vi "pmu_Simulate PMU signal.vi"(0 "physical channels":T1[](array[typedef]), 5 "elements to read":u32=250, 7 "frequency (Hz)":dbl(knob)=60.0 scale=45.0..65.0 scale format="%#.9g", 11 "error in (no error)":errorcluster) -> (4 "FIFO data":u32[](array[numeric]), 15 "error out":errorcluster)   [LabVIEW 2014]
doc: "This VI simulates pure sinewave test signal to validate the RT part of the PMU algorithm. You can set frequency, amplitude and digital signal states with this VI. This VI is intended to be used in debugging mode with its front panel open so that the user can control front panel objects."
uses:
  <vilib>/addons/Electrical Power/PMU/Common/Controls/pmu_Physical Channel.ctl
  <vilib>/addons/Electrical Power/PMU/Common/Controls/pmu_Channel Phase.ctl
  <vilib>/addons/Electrical Power/PMU/NI_EP_PMU.lvlib
panel:
  in  "Random DI":bool
  in  "DI":bool[](array[boolean])=[FALSE, FALSE, FALSE, FALSE, FALSE, FALSE, FALSE, FALSE, FALSE, FALSE, FALSE, FALSE, FALSE, FALSE, FALSE, FALSE, FALSE, FALSE, FALSE, FALSE, FALSE, FALSE, FALSE, FALSE, FALSE, FALSE, FALSE, FALSE, FALSE, FALSE, FALSE, FALSE]
  in  "current (A)":dbl(knob)=2.5 scale=0.0..5.0
  in  "voltage (V)":dbl(knob)=110.0 scale=0.0..300.0
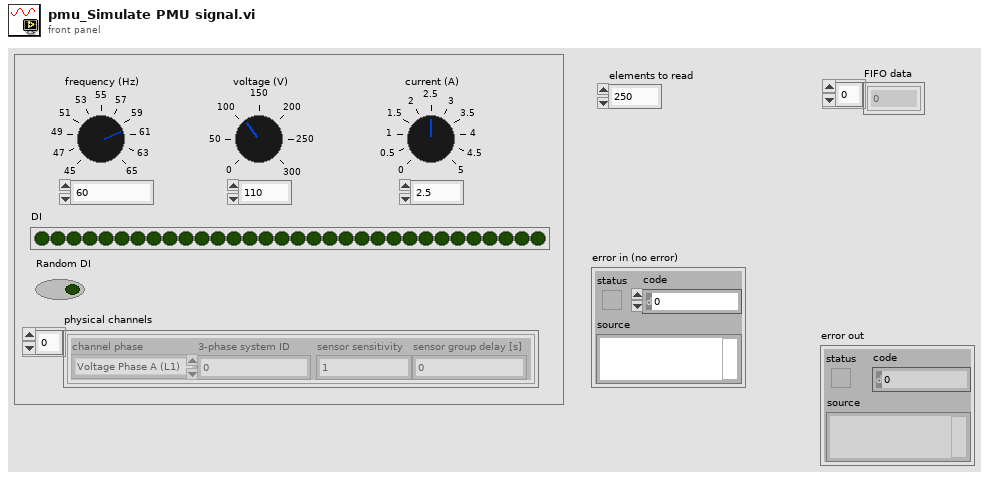
[diagram p1: front panel]
types:
  T1 = typedef "NI_EP_PMU.lvlib/pmu_Physical Channel.ctl" = cluster{"channel phase":T2, "3-phase system ID":u8, "sensor sensitivity":dbl, "sensor group delay [s]":dbl}
  T2 = typedef "NI_EP_PMU.lvlib/pmu_Channel Phase.ctl" = enum16{"Voltage Phase A (L1)", "Voltage Phase B (L2)", "Voltage Phase C (L3)", "Voltage Phase N (Neutral)", "Current Phase A (L1)", "Current Phase B (L2)", "Current Phase C (L3)", "Current Phase N (Neutral)", "Voltage Phase AB (L1L2)", "Voltage Phase BC (L2L3)", "Voltage Phase CA (L3L1)"}
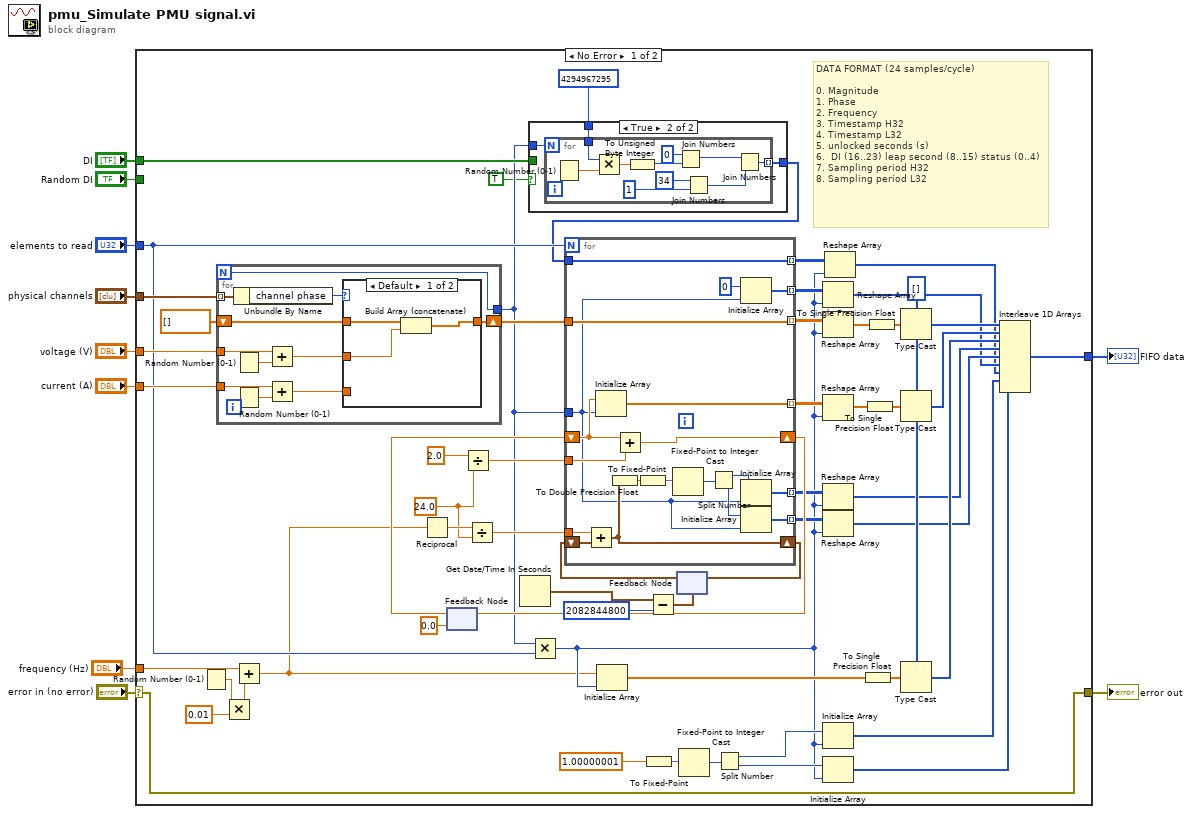
[diagram p0: block diagram]
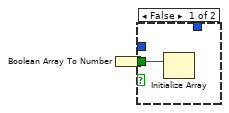
[diagram p2: hidden frame]
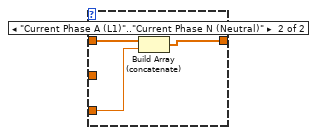
[diagram p3: hidden frame]
diagram:
  n1 = case shown="No Error" "error in (no error)" {
    selector: "error in (no error)" -> [w11 w121]
    tunnel: [w11 w121] -> w7
    tunnel: [w26 _] -> w9
    tunnel: "elements to read" -> [w50 _]
    tunnel: "voltage (V)" -> [w68 _]
    tunnel: "current (A)" -> [w67 _]
    tunnel: "frequency (Hz)" -> [w15 _]
    tunnel: "DI" -> [w62 _]
    tunnel: "Random DI" -> [_ _]
    tunnel: "physical channels" -> [w69 _]
    frame No Error {
      w48 = 24.0 ("y")
      w53 = u32[] [] ("Data")
      # "DATA FORMAT (24 samples/cycle)\n \n0. Magnitude \n1. Phase \n2. Frequency \n3. Timestamp H32 \n4. Timestamp L32 \n5. unlocked seconds (s)\n6.  DI (16..23) leap second (8..15) status (0..4)\n7. Sampling period H32\n8. Sampling period L32"
      n2 = Random Number (0-1)() -> (number: 0 to 1=w25:dbl)
      n3 = for {
        N -> [w104]
        tunnel: w69 -> [w114] mode=indexing
        shift-right: [w106] -> w63
        shift-left: dbl[] [] -> [w112]
        tunnel: w68 -> [w111]
        tunnel: w67 -> [w109]
        tunnel: [w104] -> w34
        n4 = Unbundle By Name(w114) -> ("channel phase"=w113:T2)
        n5 = Random Number (0-1)() -> (number: 0 to 1=w110:dbl)
        n6 = Random Number (0-1)() -> (number: 0 to 1=w108:dbl)
        n7 = Add(x=w111, y=w110) -> (x+y=w107:dbl)
        n8 = Add(x=w109, y=w108) -> (x+y=w105:dbl)
        n9 = case shown="Default" w113 {
          tunnel: w112 -> [w117 w119]
          tunnel: w107 -> [w116 _]
          tunnel: [w115 w118] -> w106
          tunnel: w105 -> [_ w120]
          frame Default {
            n10 = Build Array (concatenate)(w117, w116) -> (w115:dbl[])
          }
          frame "Current Phase A (L1)".."Current Phase N (Neutral)" {
            n11 = Build Array (concatenate)(w119, w120) -> (w118:dbl[])
          }
        }
      }
      n12 = Multiply(x=w25, y=0.01) -> (x*y=w23:dbl)
      n13 = Add(x=w15, y=w23) -> (x+y=w13:dbl)
      n14 = Reciprocal(x=w13) -> (1/x=w49:dbl)
      n15 = feedback #1(0.0) -> (w59:dbl)
      n16 = Divide(x=2.0 ("y"), y=w48) -> (x/y=w61:dbl)
      n17 = Divide(x=w49, y=w48) -> (x/y=w47:dbl)
      n18 = Get Date/Time In Seconds() -> (seconds since 1Jan1904=w21:timestamp)
      n19 = case shown="True" TRUE {
        tunnel: w62 -> [w71 _]
        tunnel: w34 -> [_ w74]
        tunnel: [_ w73] -> w31
        tunnel: u32 4294967295 -> [_ w72]
        frame False {
          n20 = Boolean Array To Number(Boolean array=w71) -> (number=w70:u32)
          n21 = Initialize Array(w70) -> ()  [unwired: 1 in, 1 out]
        }
        frame True {
          n22 = for {
            N: w74 -> [_]
            tunnel: [w81] -> w73 mode=indexing
            tunnel: w72 -> [w79]
            n23 = Random Number (0-1)() -> (number: 0 to 1=w80:dbl)
            n24 = Multiply(x=w79, y=w80) -> (x*y=w84:dbl)
            n25 = To Unsigned Byte Integer(number=w84) -> (unsigned 8bit integer=w78:u8)
            n26 = Join Numbers(hi=u8 0, lo=w78) -> ((hi.lo)=w82:u16)
            n27 = Join Numbers(hi=u8 34, lo=u8 1) -> ((hi.lo)=w83:u16)
            n28 = Join Numbers(hi=w82, lo=w83) -> ((hi.lo)=w81:u32)
          }
        }
      }
      n29 = Multiply(x=w34, y=w50) -> (x*y=w18:u32)
      n30 = Initialize Array(w13, w18) -> (w54:dbl[])
      n31 = To Fixed-Point(number=1.00000001 ("x/y")) -> (fixed-point=w40:fxp<+,64,32>)  [unwired: 1 in]
      n32 = Subtract(x=w21, y=u32 2082844800 ("unsigned 32bit integer")) -> (x-y=w20:timestamp)
      n33 = feedback #2(w20) -> (w51:timestamp)
      n34 = for {
        N: w50 -> [_]
        tunnel: w63 -> [w96]
        shift-right: [w102] -> w60
        shift-left: w59 -> [w101]
        tunnel: w61 -> [w103]
        tunnel: w34 -> [w87]
        shift-right: [w98] -> w52
        shift-left: w51 -> [w100]
        tunnel: w47 -> [w99]
        tunnel: [w96] -> w45 mode=indexing
        tunnel: [w95] -> w44 mode=indexing
        tunnel: [w90] -> w43 mode=indexing
        tunnel: [w89] -> w42 mode=indexing
        tunnel: w31 -> [w85]
        tunnel: [w86] -> w30 mode=indexing
        tunnel: [w85] -> w19 mode=indexing
        n35 = Add(x=w99, y=w100) -> (x+y=w98:timestamp)
        n36 = Initialize Array(w101, w87) -> (w95:dbl[])
        n37 = To Double Precision Float(number=w98) -> (double precision float=w97:dbl)
        n38 = Add(x=w101, y=w103) -> (x+y=w102:dbl)
        n39 = To Fixed-Point(number=w97) -> (fixed-point=w94:fxp<+,64,32>)  [unwired: 1 in]
        n40 = Fixed-Point to Integer Cast(1:w94) -> (0:w93:u64)
        n41 = Split Number(x=w93) -> (hi(x)=w92:u32, lo(x)=w91:u32)
        n42 = Initialize Array(u32 0 ("element"), w87) -> (w86:u32[])
        n43 = Initialize Array(w92, w87) -> (w90:u32[])
        n44 = Initialize Array(w91, w87) -> (w89:u32[])
      }
      n45 = feedback-in #1(w60) -> ()
      n46 = feedback-in #2(w52) -> ()
      n47 = Fixed-Point to Integer Cast(1:w40) -> (0:w39:u64)
      n48 = Split Number(x=w39) -> (hi(x)=w38:u32, lo(x)=w37:u32)
      n49 = Reshape Array(w30, w18) -> (w27:u32[])
      n50 = Reshape Array(w45, w18) -> (w41:dbl[])
      n51 = Reshape Array(w44, w18) -> (w33:dbl[])
      n52 = Reshape Array(w43, w18) -> (w29:u32[])
      n53 = Reshape Array(w42, w18) -> (w28:u32[])
      n54 = Initialize Array(w38, w18) -> (w35:u32[])
      n55 = Initialize Array(w37, w18) -> (w36:u32[])
      n56 = Reshape Array(w19, w18) -> (w17:u32[])
      n57 = To Single Precision Float(number=w54) -> (single precision float=w55:sgl[])
      n58 = To Single Precision Float(number=w33) -> (single precision float=w57:sgl[])
      n59 = To Single Precision Float(number=w41) -> (single precision float=w65:sgl[])
      n60 = Type Cast(type=w53, x=w65) -> (*(type *) &x=w64:u32[])
      n61 = Type Cast(type=w53, x=w57) -> (*(type *) &x=w56:u32[])
      n62 = Type Cast(type=w53, x=w55) -> (*(type *) &x=w46:u32[])
      n63 = Interleave 1D Arrays(w64, w56, w46, w29, w28, w27, w17, w35, w36) -> (w26:u32[])
    }
    frame Error {
    }
  }
  "error out" <- w7
  "FIFO data" <- w9
